vi "solar_voy_def Resolve ASCII (Default).vi"(9 "Default (NaN=Use Default)":dbl=nan, 10 "DEFAULT,MIN,MAX":string) -> (2 "DEFAULT,MIN,MAX out":dbl)   [LabVIEW 2018]
doc: "This determines the MIN, MAX or VALUE of the string input. This also handles hexidecimal '\\xFFFF' and octal '\\o6666' strings."
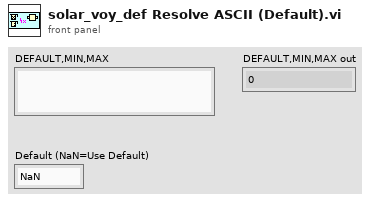
[diagram p1: front panel]
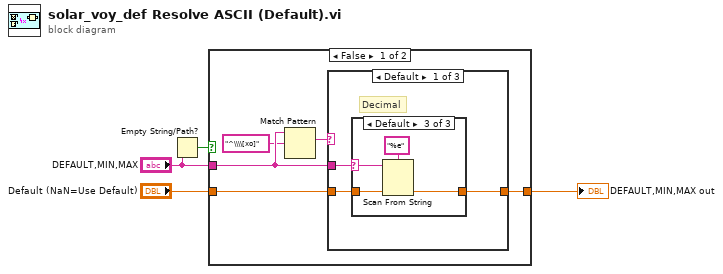
[diagram p0: block diagram]
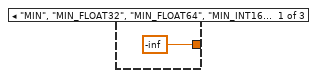
[diagram p2: hidden frame]
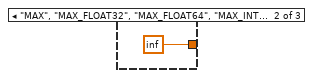
[diagram p3: hidden frame]
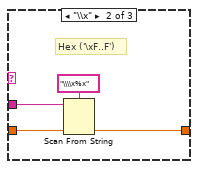
[diagram p4: hidden frame]
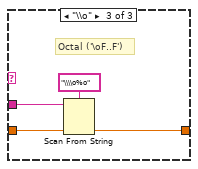
[diagram p5: hidden frame]
diagram:
  n1 = Empty String/Path?(string/path="DEFAULT,MIN,MAX") -> (empty?=w1:bool)
  n2 = case shown="False" w1 {
    tunnel: [w9 w27] -> w4
    tunnel: "Default (NaN=Use Default)" -> [w8 w27]
    tunnel: "DEFAULT,MIN,MAX" -> [w7 _]
    frame False {
      n3 = Match Pattern(string=w7, regular expression="^\\\\[xo]") -> (match substring=w5:string)  [unwired: 1 in, 3 out]
      n4 = case shown="Default" w5 {
        tunnel: [w12 w22 w26] -> w9
        tunnel: w8 -> [w11 w21 w25]
        tunnel: w7 -> [w10 w20 w24]
        frame Default {
          # "Decimal"
          n5 = case shown="Default" w10 {
            selector: w10 -> [_ _ w18]
            tunnel: w11 -> [_ _ w17]
            tunnel: [-inf ("MIN") inf ("MIN") w16] -> w12
            frame "MIN", "MIN_FLOAT32", "MIN_FLOAT64", "MIN_INT16", "MIN_INT32", "MIN_INT64", "MIN_INT8", "MIN_UINT16", "MIN_UINT32", "MIN_UINT64", "MIN_UINT8" {
            }
            frame "MAX", "MAX_FLOAT32", "MAX_FLOAT64", "MAX_INT16", "MAX_INT32", "MAX_INT64", "MAX_INT8", "MAX_UINT16", "MAX_UINT32", "MAX_UINT64", "MAX_UINT8" {
            }
            frame Default {
              n6 = Scan From String(format string="%e", input string=w18, default 1=w17) -> (output 1=w16:dbl)  [unwired: 2 in, 3 out]
            }
          }
        }
        frame "\\x" {
          # "Hex ('\\xF..F')"
          n7 = Scan From String(format string="\\\\x%x", input string=w20, default 1=w21) -> (output 1=w22:dbl)  [unwired: 2 in, 3 out]
        }
        frame "\\o" {
          # "Octal ('\\oF..F')"
          n8 = Scan From String(format string="\\\\o%o", input string=w24, default 1=w25) -> (output 1=w26:dbl)  [unwired: 2 in, 3 out]
        }
      }
    }
    frame True {
    }
  }
  "DEFAULT,MIN,MAX out" <- w4
